vi "GSP_Dialog_2Buttons.vi"(4 "error in (no error)":errorcluster, 6 "Messages (Custom)":T1, 7 "Message":string) -> (0 "error out":errorcluster, 2 "OK Button?":bool)   [LabVIEW 2015]
uses:
  dialog_messages.ctl
panel:
  in  "Cancel":bool
  in  "OK":bool
  out "String":string
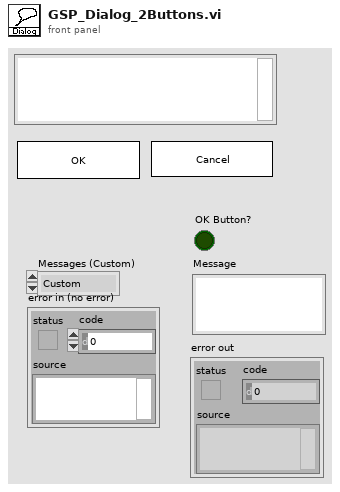
[diagram p1: front panel]
types:
  T1 = typedef "dialog_messages.ctl" = enum16{"Custom", "Incompatible Config"}
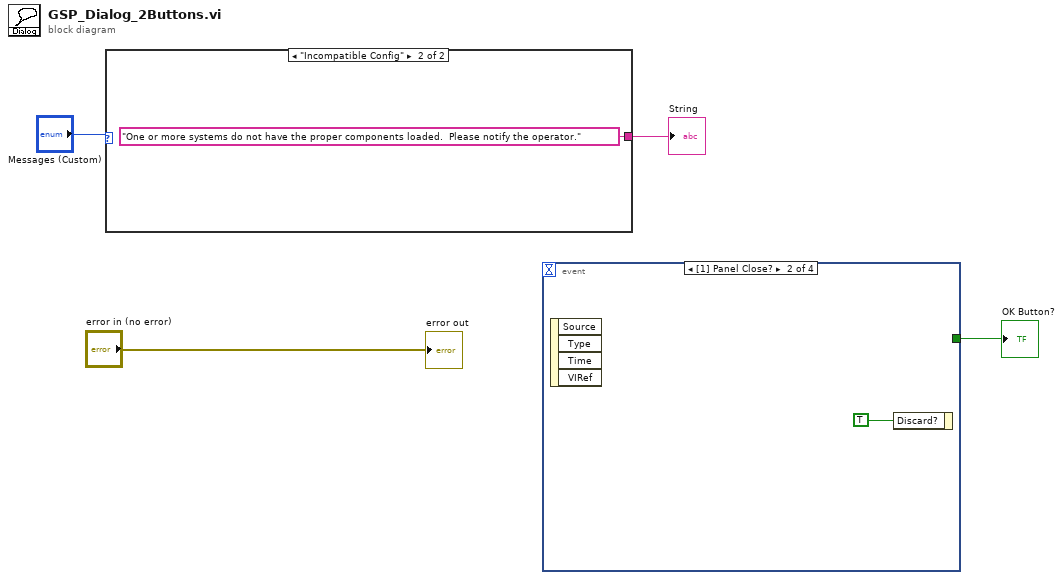
[diagram p0: block diagram]
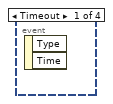
[diagram p2: hidden frame]
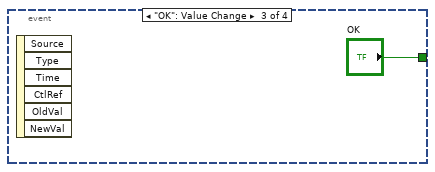
[diagram p3: hidden frame]
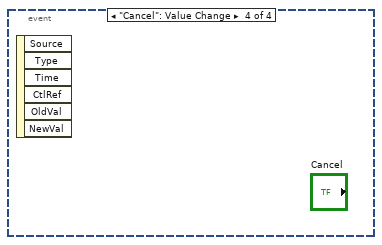
[diagram p4: hidden frame]
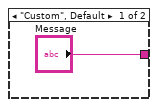
[diagram p5: hidden frame]
diagram:
  n1 = case shown="\"Incompatible Config\"" "Messages (Custom)" {
    tunnel: ["Message" "One or more systems do not have the proper components loaded.  Please notify the operator." ("Message")] -> w2
    frame "Custom", Default {
    }
    frame "Incompatible Config" {
    }
  }
  "String" <- w2
  n2 = event shown="[1] Panel Close?" {
    selector: _ -> [_ _ _ _]
    dyn-events: _ -> [_ _ _ _]
    timeout: _ -> [_ _ _ _]
    tunnel: [_ _ "OK" _] -> w1
    event Timeout {
      n3 = event-data() -> ()  [unwired: 1 in, 2 out]
    }
    event Panel Close? {
      n4 = event-data() -> ()  [unwired: 1 in, 4 out]
      n5 = event-data("Discard?"=TRUE) -> ()  [unwired: 1 in, 1 out]
    }
    event "OK": Value Change {
      n6 = event-data() -> ()  [unwired: 1 in, 6 out]
    }
    event "Cancel": Value Change {
      n7 = event-data() -> ()  [unwired: 1 in, 6 out]
    }
  }
  "OK Button?" <- w1
  "error out" <- "error in (no error)"
